vi "RWNoise-Init Timing.vi"(0 "RWN Stim":T29, 7 "RW Noise Params":T27, 11 "error in (no error)":errorcluster) -> (4 "Runtime":T1={"Stimulus"={"Waveform"={"Type"=enum."Tone", "Tone"={"Frequency (kHz)"=0.0, "Last Freq"=0.0, "Last Phase"=0.0}, "Pulse Train"={"Pulse width (us)"=0.0, "Pulse rate (Hz)"=0.0, "Gap (ms)"=0.0, "Polarity"=enum."POS", "PT State"={"Template"=[], "Nperiod"=0, "Index"=0, "Pulse Rate (Hz)"=0.0, "Phase (cycles)"=0.0, "Noff"=0}, "Asynch"=FALSE}, "Noise"={"InvFilt"=FALSE, "Noise"=[], "CurPt"=0, "Aweight"=FALSE, "Seed"=0, "afile"=path ""}, "File"={"Filename"=path "", "Signal"=[], "Channel"=0, "stream"=FALSE, "offset"=0, "nreps"=0, "loops"=0, "Randomize"=FALSE, "order"=[], "Seed"=0, "Tokens"=0}, "FMSweep"={"Rate (oct/s)"=0.0, "Fmin (Hz)"=0.0, "Fmax (Hz)"=0.0, "Ramp (ms)"=0.0, "Linear"=FALSE}, "Chirp Train"={"Params"={"Fmin (kHz)"=4.0, "Fmax (kHz)"=64.0, "Compensate"=FALSE, "Duration (ms)"=2.0}, "Data"={"WF"=[]}}, "Complex Tone"={"Params"={"F0 (Hz)"=0.0, "Band"={"Flow (Hz)"=0.0, "Fhigh (Hz)"=0.0}, "Phase"=enum."Cosine", "Min F0 (Hz)"=0.0, "Max F0 (Hz)"=0.0, "ContinRandPhase"=FALSE, "Max peak factor"=inf, "Max mod depth"=2.0, "MinHarmNum"=0, "MaxHarmNum"=0, "Level Mode"=enum."per component", "% jitter"=0.0}, "Data"={"Ncomp"=0, "MinHarm"=0, "Phase"=[], "Amplitude"=[], "Npts/frame"=0, "Last F0"=0.0, "Fmin"=0.0, "Fmax"=0.0, "Lslope"=0.0, "randphase"=FALSE, "overall rms"=FALSE, "fmult"=[], "jittered"=FALSE}}, "Moving Ripple"={"Params"={"Fmin"=0.0, "Fmax"=0.0, "Density"=0.0, "Velocity"=0.0, "Depth"=0.0, "Phase"=0.0, "Comp/oct"=0}, "Data"={"Freq"=[], "A"=[], "phase"=[], "Phase"=0.0}}}, "Filter"={"Type"=enum."Lowpass", "CF (kHz)"=0.0, "BW (kHz)"=0.0, "Cascade"=FALSE, "Quadrature"=FALSE, "Scale Factor"=0.0, "Stages"=[], "Class"=enum."Elliptic", "Order"=0, "BWUnits"=enum."Linear"}, "Burst"={"Active"=FALSE, "Delay (ms)"=0.0, "Duration (ms)"=0.0, "Ramp (ms)"=0.0, "Rate (Hz)"=0.0, "Trepeat (ms)"=0.0, "Repeat"=FALSE}, "Level"={"Level"=0.0, "Units"=enum."dB atten", "Max"=0.0, "Multiplier"=0.0, "Cal File"=path "", "Cal"={"Freq (Hz)"=[], "Mag (dB SPL)"=[], "Phase (deg)"=[]}}, "Name"="", "Advanced"={"Rep Mask"="", "AltPol"=FALSE, "Var"="", "Expr"="", "Persist"=FALSE}, "SAM"={"Active"=FALSE, "Frequency (Hz)"=0.0, "Depth"=0.0, "Init Phase (cycles)"=0.0, "phase (degrees)"=0.0, "Asynch"=FALSE}}, "Fs (Hz)"=0.0, "AO Npts"=0, "AO Channels"=[], "Active"=FALSE, "AINpts"=0, "WinPts"=0, "NUpdate"=0} {"Stimulus"."Filter"."Stages"."IIR Filter"."Forward Coefficients" format="%.4f"; "Stimulus"."Filter"."Stages"."IIR Filter"."Reverse Coefficients" format="%.4f"}, 8 "Burst Params":T22={"Active"=FALSE, "Delay (ms)"=0.0, "Duration (ms)"=50.0, "Ramp (ms)"=5.0, "Rate (Hz)"=0.0, "Trepeat (ms)"=0.0, "Repeat"=FALSE}, 15 "error out":errorcluster)   [LabVIEW 2020]
uses:
  RWNoise-Stim Params.ctl
  RWNoise Params.ctl
  epl-vi-lib/Utility VIs/Type Defs/Left-Right ring.ctl
  epl-vi-lib/Signal Synthesis VIs/Controls/Burst XCtl/Burst Data.ctl
  RWNoise-Runtime Data.ctl
  epl-vi-lib/Signal Synthesis VIs/Controls/Stimulus Channel (Full)/Full Stimulus Channel Data.ctl
  epl-vi-lib/Signal Synthesis VIs/Controls/Waveform XCtl/Waveform Data.ctl
  epl-vi-lib/Signal Synthesis VIs/Controls/Waveform XCtl/Waveform Enum.ctl
  epl-vi-lib/Signal Synthesis VIs/Waveform VIs/Tone VIs/Tone Params.ctl
  epl-vi-lib/Signal Synthesis VIs/Waveform VIs/Pulse Train VIs/Pulse Train Params.ctl
  epl-vi-lib/Signal Synthesis VIs/Waveform VIs/Pulse Train VIs/Pulse Polarity.ctl
  epl-vi-lib/Signal Synthesis VIs/Waveform VIs/Pulse Train VIs/PT-Continuous State.ctl
  epl-vi-lib/Signal Synthesis VIs/Waveform VIs/Noise VIs/Noise Params.ctl
  epl-vi-lib/Signal Synthesis VIs/Waveform VIs/File VIs/StimFile-Params.ctl
  epl-vi-lib/Signal Synthesis VIs/Waveform VIs/FM Sweep VIs/FM Sweep Params.ctl
  epl-vi-lib/Signal Synthesis VIs/Waveform VIs/Chirp Train VIs/Chirp Train.ctl
  epl-vi-lib/Signal Synthesis VIs/Waveform VIs/Chirp Train VIs/Chirp Train Params.ctl
  epl-vi-lib/Signal Synthesis VIs/Waveform VIs/Complex Tone VIs/CT-Params.ctl
  epl-vi-lib/Signal Synthesis VIs/Waveform VIs/Complex Tone VIs/CT-Phase Enum.ctl
  epl-vi-lib/Signal Synthesis VIs/Waveform VIs/Complex Tone VIs/CT-Runtime Data.ctl
  epl-vi-lib/Signal Synthesis VIs/Waveform VIs/Moving Ripple VIs/Moving Ripple.ctl
  epl-vi-lib/Signal Synthesis VIs/Waveform VIs/Moving Ripple VIs/Moving Ripple.Params.ctl
  epl-vi-lib/Signal Synthesis VIs/Waveform VIs/Moving Ripple VIs/Moving Ripple.Data.ctl
  epl-vi-lib/Signal Synthesis VIs/Controls/Advanced Filter XCtl/Filter Data.ctl
  epl-vi-lib/Signal Synthesis VIs/Filter VIs/Filter-Bandwidth Units.ctl
  epl-vi-lib/Signal Synthesis VIs/Controls/Level XCtl/Level Data.ctl
  epl-vi-lib/Signal Synthesis VIs/Controls/Level XCtl/Level Units.ctl
  epl-vi-lib/Signal Synthesis VIs/Controls/Advanced Options XCtl/Advanced Stimulus Options.ctl
  epl-vi-lib/Signal Synthesis VIs/Modulation VIs/SAM VIs/SAM Params.ctl
  epl-vi-lib/Signal Synthesis VIs/Controls/Burst XCtl/Burst Control.xctl
  epl-vi-lib/Signal Synthesis VIs/Controls/Advanced Filter XCtl/Advanced Filter XCtl.xctl
  epl-vi-lib/Signal Synthesis VIs/Controls/Level XCtl/Level XCtl.xctl
  epl-vi-lib/Signal Synthesis VIs/Controls/Waveform XCtl/Waveform XCtl.xctl
  epl-vi-lib/Signal Synthesis VIs/Controls/Advanced Options XCtl/Advanced Stimulus Options.xctl
  epl-vi-lib/Signal Synthesis VIs/Controls/Stimulus Channel (Full)/Stimulus Channel (Full).xctl
panel:
  in  "AO Fs (Hz)":dbl=100000.0
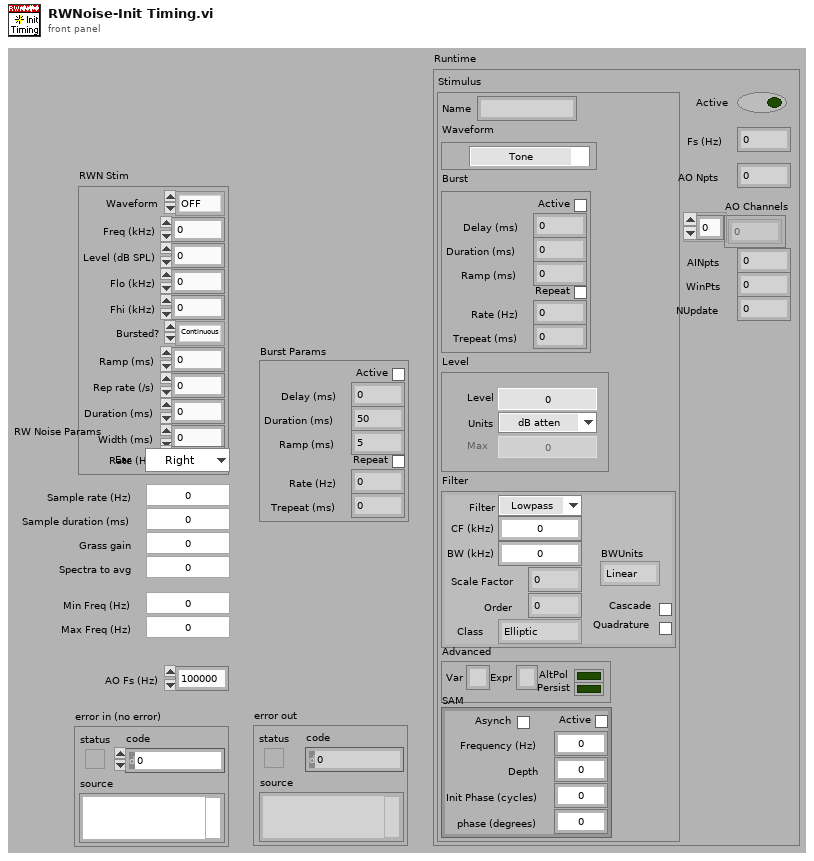
[diagram p1: front panel]
types:
  T1 = typedef "RWNoise-Runtime Data.ctl" = cluster{"Stimulus":T2, "Fs (Hz)":dbl, "AO Npts":i32, "AO Channels":i32[], "Active":bool, "AINpts":i32, "WinPts":i32, "NUpdate":i32}
  T2 = typedef "Stimulus Channel (Full).xctl/Full Stimulus Channel Data.ctl" = cluster{"Waveform":T3, "Filter":T20, "Burst":T22, "Level":T23, "Name":string, "Advanced":T25, "SAM":T26}
  T3 = typedef "Waveform XCtl.xctl/Waveform Data.ctl" = cluster{"Type":T4, "Tone":T5, "Pulse Train":T6, "Noise":T9, "File":T10, "FMSweep":T11, "Chirp Train":T12, "Complex Tone":cluster{"Params":T14, "Data":T16}, "Moving Ripple":T17}
  T4 = typedef "Waveform Enum.ctl" = enum16{"OFF", "Tone", "Noise", "Pulse Train", "File", "FM Sweep", "Chirp Train", "Complex Tone", "FM Tone", "Moving Ripple"}
  T5 = typedef "Tone Params.ctl" = cluster{"Frequency (kHz)":dbl, "Last Freq":dbl, "Last Phase":dbl}
  T6 = typedef "Pulse Train Params.ctl" = cluster{"Pulse width (us)":dbl, "Pulse rate (Hz)":dbl, "Gap (ms)":dbl, "Polarity":T7, "PT State":T8, "Asynch":bool}
  T7 = typedef "Pulse Polarity.ctl" = enum16{"POS", "NEG", "POS-NEG", "NEG-POS"}
  T8 = typedef "PT-Continuous State.ctl" = cluster{"Template":dbl[], "Nperiod":i32, "Index":i32, "Pulse Rate (Hz)":dbl, "Phase (cycles)":dbl, "Noff":i32}
  T9 = typedef "Noise Params.ctl" = cluster{"InvFilt":bool, "Noise":dbl[], "CurPt":i32, "Aweight":bool, "Seed":i32, "afile":path}
  T10 = typedef "StimFile-Params.ctl" = cluster{"Filename":path, "Signal":dbl[], "Channel":i32, "stream":bool, "offset":i32, "nreps":i32, "loops":i32, "Randomize":bool, "order":i32[], "Seed":i32, "Tokens":i32}
  T11 = typedef "FM Sweep Params.ctl" = cluster{"Rate (oct/s)":dbl, "Fmin (Hz)":dbl, "Fmax (Hz)":dbl, "Ramp (ms)":dbl, "Linear":bool}
  T12 = typedef "Chirp Train.ctl" = cluster{"Params":T13, "Data":cluster{"WF":dbl[]}}
  T13 = typedef "Chirp Train Params.ctl" = cluster{"Fmin (kHz)":dbl, "Fmax (kHz)":dbl, "Compensate":bool, "Duration (ms)":dbl}
  T14 = typedef "CT-Params.ctl" = cluster{"F0 (Hz)":dbl, "Band":cluster{"Flow (Hz)":dbl, "Fhigh (Hz)":dbl}, "Phase":T15, "Min F0 (Hz)":dbl, "Max F0 (Hz)":dbl, "ContinRandPhase":bool, "Max peak factor":dbl, "Max mod depth":dbl, "MinHarmNum":i32, "MaxHarmNum":i32, "Level Mode":enum16{"per component", "overall rms"}, "% jitter":dbl}
  T15 = typedef "CT-Phase Enum.ctl" = enum16{"Cosine", "Random", "Alternating"}
  T16 = typedef "CT-Runtime Data.ctl" = cluster{"Ncomp":i32, "MinHarm":i32, "Phase":dbl[], "Amplitude":dbl[], "Npts/frame":i32, "Last F0":dbl, "Fmin":dbl, "Fmax":dbl, "Lslope":dbl, "randphase":bool, "overall rms":bool, "fmult":dbl[], "jittered":bool}
  T17 = typedef "Moving Ripple.ctl" = cluster{"Params":T18, "Data":T19}
  T18 = typedef "Moving Ripple.Params.ctl" = cluster{"Fmin":dbl, "Fmax":dbl, "Density":dbl, "Velocity":dbl, "Depth":dbl, "Phase":dbl, "Comp/oct":i32}
  T19 = typedef "Moving Ripple.Data.ctl" = cluster{"Freq":dbl[], "A":dbl[], "phase":dbl[], "Phase":dbl}
  T20 = typedef "Advanced Filter XCtl.xctl/Filter Data.ctl" = cluster{"Type":enum16{"Lowpass", "Highpass", "Bandpass", "Bandstop", "OFF"}, "CF (kHz)":dbl, "BW (kHz)":dbl, "Cascade":bool, "Quadrature":bool, "Scale Factor":dbl, "Stages":cluster{"IIR Filter":cluster{"filter structure":enum32{"IIR 2nd Order", "IIR 4th Order"}, "Reverse Coefficients":dbl[], "Forward Coefficients":dbl[]}, "State":dbl[]}[], "Class":enum16{"Elliptic", "Butterworth"}, "Order":i32, "BWUnits":T21}
  T21 = typedef "Filter-Bandwidth Units.ctl" = enum16{"Linear", "Octaves", "Min-Max"}
  T22 = typedef "Burst Control.xctl/Burst Data.ctl" = cluster{"Active":bool, "Delay (ms)":dbl, "Duration (ms)":dbl, "Ramp (ms)":dbl, "Rate (Hz)":dbl, "Trepeat (ms)":dbl, "Repeat":bool}
  T23 = typedef "Level XCtl.xctl/Level Data.ctl" = cluster{"Level":dbl, "Units":T24, "Max":dbl, "Multiplier":dbl, "Cal File":path, "Cal":cluster{"Freq (Hz)":dbl[], "Mag (dB SPL)":dbl[], "Phase (deg)":dbl[]}}
  T24 = typedef "Level Units.ctl" = enum16{"dB atten", "dB SPL", "dB re 1 Vrms", "dB V/Hz½", "mW", "dB HL", "Volts", "dB mW"}
  T25 = typedef "Advanced Stimulus Options.xctl/Advanced Stimulus Options.ctl" = cluster{"Rep Mask":string, "AltPol":bool, "Var":string, "Expr":string, "Persist":bool}
  T26 = typedef "SAM Params.ctl" = cluster{"Active":bool, "Frequency (Hz)":dbl, "Depth":dbl, "Init Phase (cycles)":dbl, "phase (degrees)":dbl, "Asynch":bool}
  T27 = typedef "RWNoise Params.ctl" = cluster{"Sample rate (Hz)":dbl, "Sample duration (ms)":dbl, "Grass gain":dbl, "Min Freq (Hz)":dbl, "Max Freq (Hz)":dbl, "Spectra to avg":i32, "Ear":T28}
  T28 = typedef "Left-Right ring.ctl" = enum16{"Right", "Left"}
  T29 = typedef "RWNoise-Stim Params.ctl" = cluster{"Waveform":enum16{"OFF", "Tone", "Noise", "Pulses"}, "Freq (kHz)":dbl, "Level (dB SPL)":dbl, "Flo (kHz)":dbl, "Fhi (kHz)":dbl, "Ramp (ms)":dbl, "Rep rate (/s)":dbl, "Bursted?":enum16{"Continuous", "Bursted"}, "Duration (ms)":dbl, "Width (ms)":dbl, "Rate (Hz)":dbl}
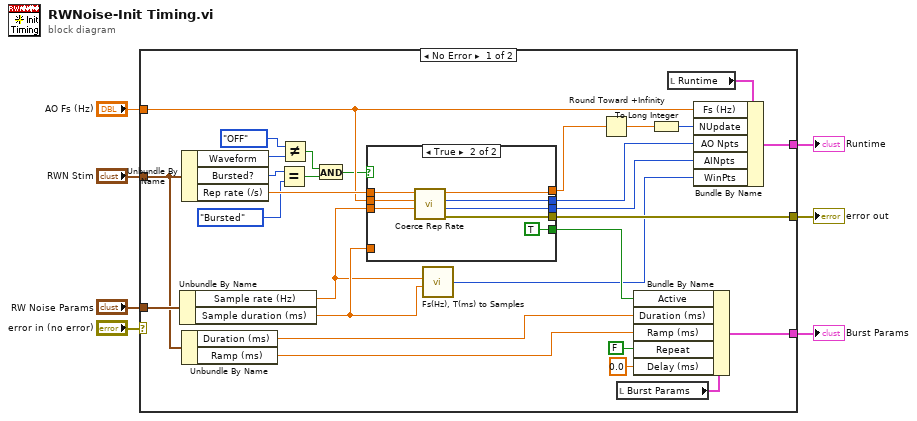
[diagram p0: block diagram]
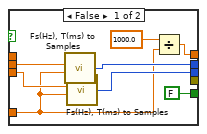
[diagram p2: hidden frame]
diagram:
  n1 = case shown="No Error" "error in (no error)" {
    selector: "error in (no error)" -> [_ w53]
    tunnel: "RWN Stim" -> [w30 _]
    tunnel: "RW Noise Params" -> [w36 _]
    tunnel: "AO Fs (Hz)" -> [w26 _]
    tunnel: [w31 _] -> w3
    tunnel: [w22 w53] -> w2
    tunnel: [w23 _] -> w1
    frame No Error {
      n2 = Unbundle By Name(w36) -> ("Sample rate (Hz)"=w20:dbl, "Sample duration (ms)"=w21:dbl)
      n3 = Unbundle By Name(w30) -> ("Waveform"=w18:enum16{"OFF", "Tone", "Noise", "Pulses"}, "Bursted?"=w14:enum16{"Continuous", "Bursted"}, "Rep rate (/s)"=w32:dbl)
      n4 = Unbundle By Name(w30) -> ("Duration (ms)"=w8:dbl, "Ramp (ms)"=w29:dbl)
      n5 = Equal?(x=w14, y=enum16{"Continuous", "Bursted"}."Bursted") -> (x = y?=w13:bool)
      n6 = Not Equal?(x=enum16{"OFF", "Tone", "Noise"}."OFF", y=w18) -> (x != y?=w16:bool)
      n7 = And(x=w16, y=w13) -> (x .and. y?=w15:bool)
      n8 = case shown="True" w15 {
        tunnel: [FALSE TRUE] -> w28
        tunnel: w32 -> [_ w51]
        tunnel: w26 -> [w43 w50]
        tunnel: w20 -> [w41 w49]
        tunnel: [w42 w48] -> w25
        tunnel: [w40 w47] -> w24
        tunnel: w21 -> [w38 _]
        tunnel: [_ w46] -> w22
        tunnel: [w39 w45] -> w11
        frame False {
          n9 = call "Fs(Hz), T(ms) to Samples.vi"("Duration (ms)"=w38, "Sampling rate (Hz)"=w43) -> ("Samples"=w42:i32)  [unwired: 4 in]
          n10 = call "Fs(Hz), T(ms) to Samples.vi"("Duration (ms)"=w38, "Sampling rate (Hz)"=w41) -> ("Samples"=w40:i32)  [unwired: 4 in]
          n11 = Divide(x=1000.0, y=w38) -> (x/y=w39:dbl)
        }
        frame True {
          n12 = call "Coerce Rep Rate.vi"("AI sampling rate (Hz)"=w49, "AO sampling rate (Hz)"=w50, "Rep rate (Hz)"=w51) -> ("error out"=w46:errorcluster, "AI npts"=w47:i32, "AO npts"=w48:i32, "Coerced rep rate (Hz)"=w45:dbl)  [unwired: 5 in]
        }
      }
      n13 = call "Fs(Hz), T(ms) to Samples.vi"("Duration (ms)"=w21, "Sampling rate (Hz)"=w20) -> ("Samples"=w19:i32)  [unwired: 4 in]
      n14 = Round Toward +Infinity(x=w11) -> (ceil(x): smallest int >= x=w9:dbl)
      n15 = local read "Burst Params"() -> (w35:T22)
      n16 = Bundle By Name(cluster=w35, "Active"=w28, "Duration (ms)"=w8, "Ramp (ms)"=w29, "Repeat"=FALSE, "Delay (ms)"=0.0) -> (w31:T22)
      n17 = To Long Integer(number=w9) -> (32bit integer=w10:i32)
      n18 = local read "Runtime"() -> (w27:T1)
      n19 = Bundle By Name(cluster=w27, "Fs (Hz)"=w26, "NUpdate"=w10, "AO Npts"=w25, "AINpts"=w24, "WinPts"=w19) -> (w23:T1)
    }
    frame Error {
    }
  }
  "error out" <- w2
  "Burst Params" <- w3
  "Runtime" <- w1
